vi "GoToHeightWhenDriveAtDistance.vi"(6 "Synchronization":enum16{"Start", "Wait"}(ring), 7 "Description":string, 8 "Command Info In":T1, 10 "DistanceFromEnd":dbl, 11 "Height":dbl) -> (0 "Command Info Out":T1)   [LabVIEW 2018]
doc: "This template has a parameter to control whether it waits for the command to complete or not. This is useful for operations that have a timed duration or a sensor-based duration. \n\nBe sure to right-click and select New from Template and save with a new command name."
uses:
  <vilib>/Rock Robotics/WPI/Framework/Command Status Info.ctl
  <vilib>/Rock Robotics/WPI/Framework/Completion Status.ctl
  <vilib>/Rock Robotics/WPI/Framework/Completion Notifier.ctl
  Implementation/Elevator Setpoints.ctl
  Implementation/Elevator Operations.ctl
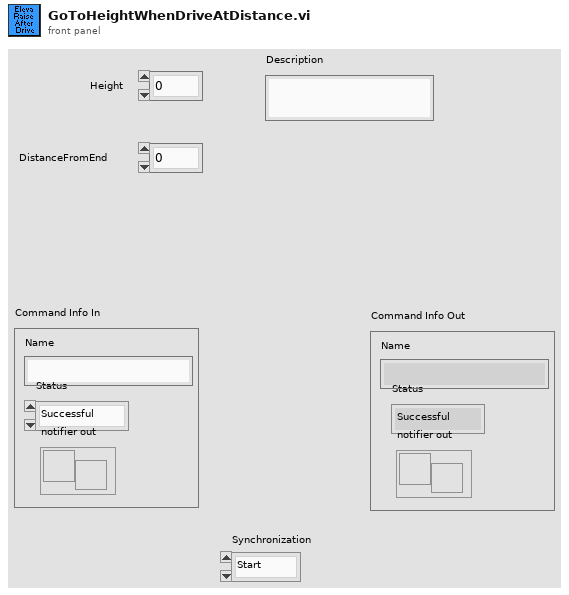
[diagram p1: front panel]
types:
  T1 = typedef "Command Status Info.ctl" = cluster{"Name":string, "Status":T2, "notifier out":T3}
  T2 = typedef "Completion Status.ctl" = enum16{"Successful", "Aborted", "Incomplete"}
  T3 = typedef "Completion Notifier.ctl" = refnum<notifier>
  T4 = typedef "Elevator Operations.ctl" = enum16{"Reserve", "Read Current", "Immediate", "GoToHeight", "StayAtHeight", "LiftForTime", "HeightAfterDriveAtDist", "HeightAfterTime"}
  T5 = typedef "Elevator Setpoints.ctl" = cluster{"Operation":T4, "Setpoint":dbl, "Duration":dbl, "Button":bool, "DistanceFromEnd":dbl}
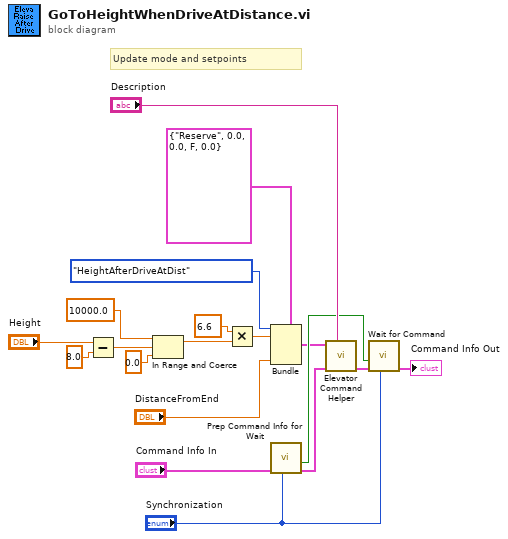
[diagram p0: block diagram]
diagram:
  # "Update mode and setpoints"
  n1 = Subtract(x="Height", y=8.0) -> (x-y=w6:dbl)
  n2 = In Range and Coerce(upper limit=10000.0, x=w6, lower limit=0.0) -> (coerced(x)=w3:dbl)  [unwired: 1 out]
  n3 = Multiply(x=6.6, y=w3) -> (x*y=w1:dbl)
  n4 = Bundle(cluster=T5 {"Operation"=enum."Reserve", "Setpoint"=0.0, "Duration"=0.0, "Button"=FALSE, "DistanceFromEnd"=0.0} ("SubSystem Data"), "Operation"=Elevator_Operations."HeightAfterDriveAtDist", "Setpoint"=w1, "DistanceFromEnd"="DistanceFromEnd") -> (w12:T5)  [unwired: 2 in]
  n5 = call <vilib>:"Prep Command Info for Wait.vi"("Synchronication"="Synchronization", "Command Info"="Command Info In") -> ("Command Info"=w16:T1, "Allocated"=w17:bool)  [unwired: 8 in]
  n6 = call "Elevator Command Helper.vi"("Description"="Description", "Command Info In"=w16, "SubSystem Data"=w12) -> ("Command Info Out"=w13:T1)  [unwired: 6 in, 2 out]
  n7 = call <vilib>:"Wait for Command.vi"("Synchronication"="Synchronization", "Command Info in"=w13, "Allocated"=w17) -> ("Command Info out"=→"Command Info Out":T1)  [unwired: 8 in]
